vi "LJM_eWriteNameArray.vi"(0 "Handle In":i32, 5 "Name":string, 9 "aValues":dbl[](array[numeric]) format="%.2f", 11 "error in":errorcluster, 13 "NumValues":i32) -> (4 "Handle Out":i32, 14 "ErrorAddress":i32, 15 "error out":errorcluster)   [LabVIEW 2020]
uses:
  Library/Frameworks/LabJackM.framework
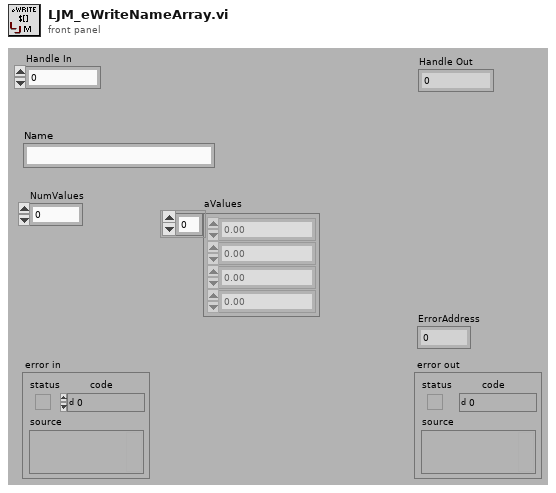
[diagram p1: front panel]
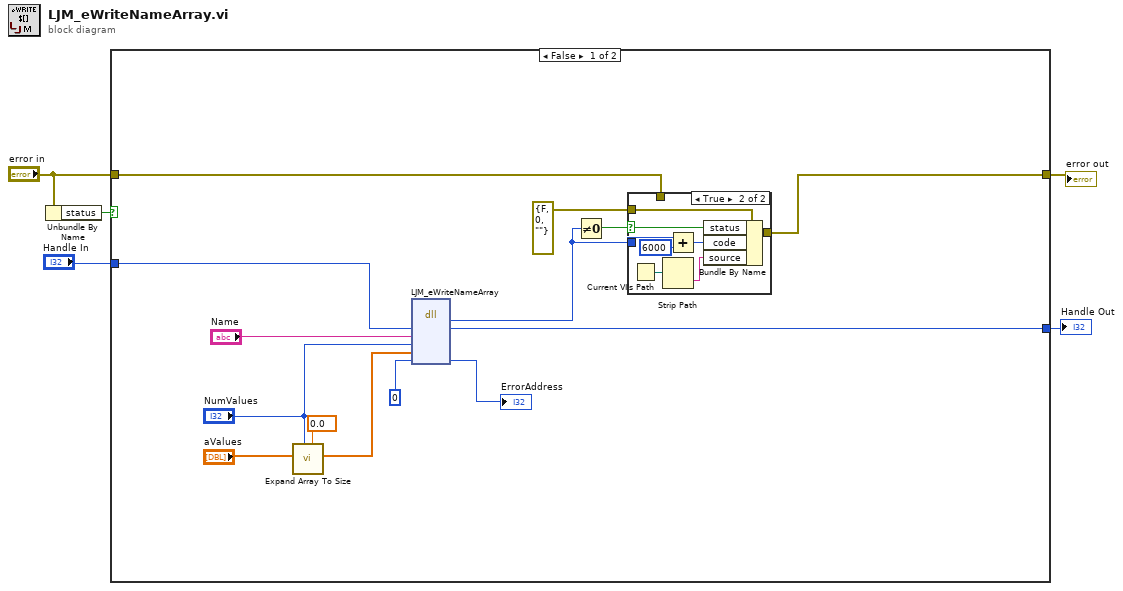
[diagram p0: block diagram]
diagram:
  n1 = Unbundle By Name("error in") -> ("status"=w2:bool)
  n2 = case shown="False" w2 {
    tunnel: "error in" -> [w16 w30]
    tunnel: [w15 w30] -> w4
    tunnel: "Handle In" -> [w14 w29]
    tunnel: [w13 w29] -> w3
    frame False {
      n3 = call "Expand Array To Size.vi"("Default Value"=0.0, "# Elements"="NumValues", "DBL Array In"="aValues") -> ("DBL Array Out"=w8:dbl[])  [unwired: 4 in, 4 out]
      n4 = dll-call lib="Library/Frameworks/LabJackM.framework" fn="LJM_eWriteNameArray"("Handle"=w14, "Name"="Name", "NumValues"="NumValues", "aValues"=w8, "ErrorAddress"=u32 0 ("ErrorFrame")) -> ("return type"=w19:i32, "Handle"=w13:i32, "ErrorAddress"=→"ErrorAddress":i32)  [unwired: 6 in, 2 out]
      n5 = Not Equal To 0?(x=w19) -> (x != 0?=w18:bool)
      n6 = case shown="True" w18 {
        selector: w18 -> [_ w27]
        tunnel: [w20 w28] -> w15
        tunnel: errorcluster {"status"=FALSE, "code"=0, "source"=""} ("error IO") -> [_ w26]
        tunnel: w19 -> [_ w22]
        tunnel: w16 -> [w20 _]
        frame False {
        }
        frame True {
          n7 = Current VI's Path() -> (path=w24:path)
          n8 = Strip Path(path=w24) -> (name=w25:string)  [unwired: 1 out]
          n9 = Add(x=w22, y=6000) -> (x+y=w23:i32)
          n10 = Bundle By Name(cluster=w26, "status"=w27, "code"=w23, "source"=w25) -> (w28:errorcluster)
        }
      }
    }
    frame True {
    }
  }
  "error out" <- w4
  "Handle Out" <- w3
